vi "Ini_Modbus.vi"(8 "error in":errorcluster, 10 "RS485 section":string="Modbus", 11 "INI file path":path=path "C:/Users/User/Desktop/YDX701_TDC/iniData/TDC_IniData.ini") -> (0 "SetCOM":bool, 1 "Parity":i32, 2 "Baud Rate":u32, 3 "COM":refnum<visa-resource-name>, 4 "ShowPlot":bool)   [LabVIEW 2019]
uses:
  <vilib>/Utility/config.llb/Read Key (String).vi
  <vilib>/Utility/config.llb/Read Key (U32).vi
  <vilib>/Utility/config.llb/Read Key (Boolean).vi
  <vilib>/Utility/config.llb/NI_LVConfig.lvlib
panel:
  out "error out":errorcluster
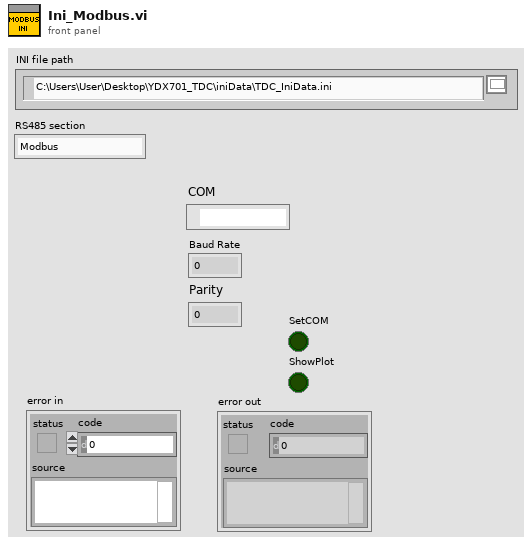
[diagram p1: front panel]
types:
  T1 = typedef "NI_LVConfig.lvlib/Config Data RefNum.ctl" = refnum<k1>
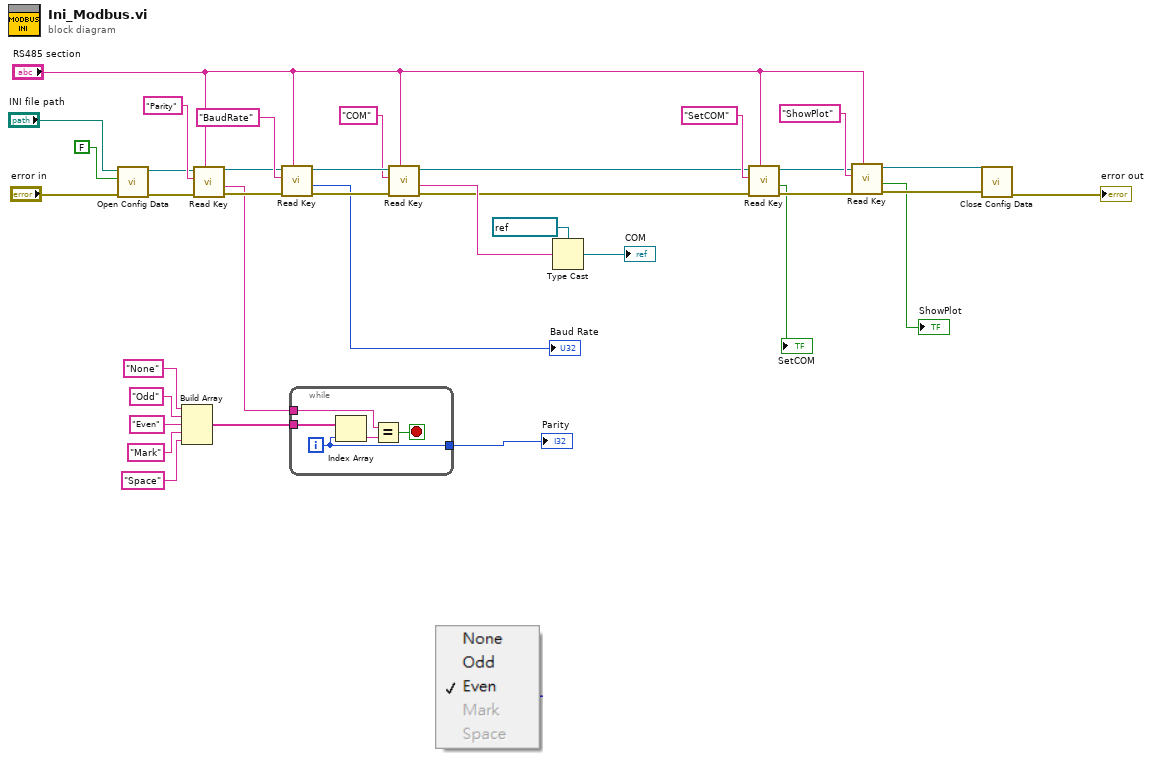
[diagram p0: block diagram]
diagram:
  n1 = call <vilib>:"Open Config Data.vi"("error in (no error)"="error in", "create file if necessary (T)"=FALSE ("create file if necessary? (T)"), "configuration file path"="INI file path") -> ("error out"=w34:errorcluster, "refnum"=w32:T1)  [unwired: 6 in, 1 out]
  n2 = Build Array("None", "Odd", "Even", "Mark", "Space") -> (w15:string[])
  n3 = call-poly <vilib>:"Read Key.vi"("section"="RS485 section", "error in (no error)"=w34, "key"="Parity", "refnum"=w32) -> ("error out"=w27:errorcluster, "value"=w14:string, "refnum out"=w28:T1)  [unwired: 2 in, 3 out]
  n4 = call-poly <vilib>:"Read Key.vi"("section"="RS485 section", "error in (no error)"=w27, "key"="BaudRate", "refnum"=w28) -> ("error out"=w25:errorcluster, "value"=→"Baud Rate":u32, "refnum out"=w26:T1)  [unwired: 1 in, 4 out]
  n5 = while {
    tunnel: w14 -> [w40]
    tunnel: w15 -> [w41]
    tunnel: [w37] -> w13
    i -> [w37]
    stop <- w38 stop-if-true
    n6 = Index Array(array=w41, index=w37) -> (element=w39:string)
    n7 = Equal?(x=w40, y=w39) -> (x = y?=w38:bool)
  }
  "Parity" <- w13
  n8 = call-poly <vilib>:"Read Key.vi"("section"="RS485 section", "error in (no error)"=w25, "key"="COM", "refnum"=w26) -> ("error out"=w9:errorcluster, "value"=w23:string, "refnum out"=w10:T1)  [unwired: 2 in, 3 out]
  n9 = Type Cast(type=refnum<visa-resource-name> "COM4" ("VISA resource name"), x=w23) -> (*(type *) &x=→"COM":refnum<visa-resource-name>)
  n10 = call-poly <vilib>:"Read Key.vi"("section"="RS485 section", "error in (no error)"=w9, "key"="SetCOM", "refnum"=w10) -> ("error out"=w6:errorcluster, "value"=→"SetCOM":bool, "refnum out"=w7:T1)  [unwired: 1 in, 4 out]
  n11 = call-poly <vilib>:"Read Key.vi"("section"="RS485 section", "error in (no error)"=w6, "key"="ShowPlot", "refnum"=w7) -> ("error out"=w4:errorcluster, "value"=→"ShowPlot":bool, "refnum out"=w5:T1)  [unwired: 1 in, 4 out]
  n12 = call <vilib>:"Close Config Data.vi"("error in (no error)"=w4, "refnum"=w5) -> ("error out"=→"error out":errorcluster)  [unwired: 1 in, 8 out]
